vi "PicoScopeospaSetDataBuffers.vi"(5 "enabled array":i16[](array[numeric]), 7 "Buffer and Transfer Settings":T3={"startIndex"=0, "Samples"=1000, "Down Sample Ratio"=1, "Down-Sample Mode"=1} {"Down-Sample Mode" items=["RAW none"=2147483648, "None"=0, "Aggregate"=1, "Decimate"=2, "Average"=4]; "Down Sample Ratio" step=1; "Samples" format="%_6p"}, 8 "error in (no error)":errorcluster, 9 "Device Info":T1, 10 "Data Pointers In":T2={"Max Buffer Pointers"=[], "Min Buffer Pointers"=[], "StreamingDataInfo"=[[{"Channel"=0, "Down-Sample Mode"=0, "PICO_DATA_TYPE"=enum."PICO_INT16_T", "Samples"=0, "bufferIndex"=0, "startIndex"=0, "overflow"=0}]]}, 11 "handle in":i16) -> (0 "error out":errorcluster, 3 "handle out":i16)   [LabVIEW 2024]
doc: "Calls SetDataBuffers, and assigns Pico buffers"
uses:
  shared/Buffer and Transfer Settings.ctl
  shared/PicoBuffers.ctl
  psospa.dll
panel:
  out "Actionflag":bool
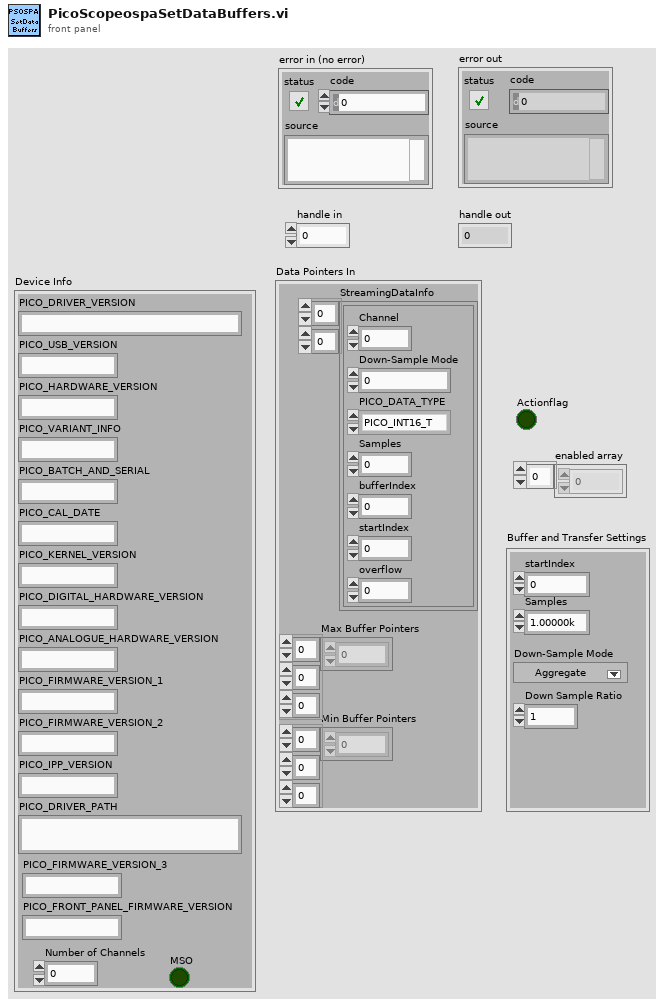
[diagram p1: front panel]
types:
  T1 = cluster{"PICO_DRIVER_VERSION":string, "PICO_USB_VERSION":string, "PICO_HARDWARE_VERSION":string, "PICO_VARIANT_INFO":string, "PICO_BATCH_AND_SERIAL":string, "PICO_CAL_DATE":string, "PICO_KERNEL_VERSION":string, "PICO_DIGITAL_HARDWARE_VERSION":string, "PICO_ANALOGUE_HARDWARE_VERSION":string, "PICO_FIRMWARE_VERSION_1":string, "PICO_FIRMWARE_VERSION_2":string, "PICO_IPP_VERSION":string, "PICO_DRIVER_PATH":string, "PICO_FIRMWARE_VERSION_3":string, "PICO_FRONT_PANEL_FIRMWARE_VERSION":string, "Number of Channels":i16, "MSO":bool}
  T2 = typedef "PicoBuffers.ctl" = cluster{"Max Buffer Pointers":u64[][][], "Min Buffer Pointers":u64[][][], "StreamingDataInfo":cluster{"Channel":u32, "Down-Sample Mode":u32, "PICO_DATA_TYPE":enum32{"PICO_INT8_T", "PICO_INT16_T", "PICO_INT32_T", "PICO_UINT32_T", "PICO_INT64_T", ""}, "Samples":i32, "bufferIndex":u64, "startIndex":i32, "overflow":i16}[][]}
  T3 = typedef "Buffer and Transfer Settings.ctl" = cluster{"startIndex":u64, "Samples":u64, "Down Sample Ratio":u64, "Down-Sample Mode":u32}
  T4 = enum32{"PICO_INT8_T", "PICO_INT16_T", "PICO_INT32_T", "PICO_UINT32_T", "PICO_INT64_T", ""}
  T5 = cluster{"status":bool, "code":u32, "source":string}
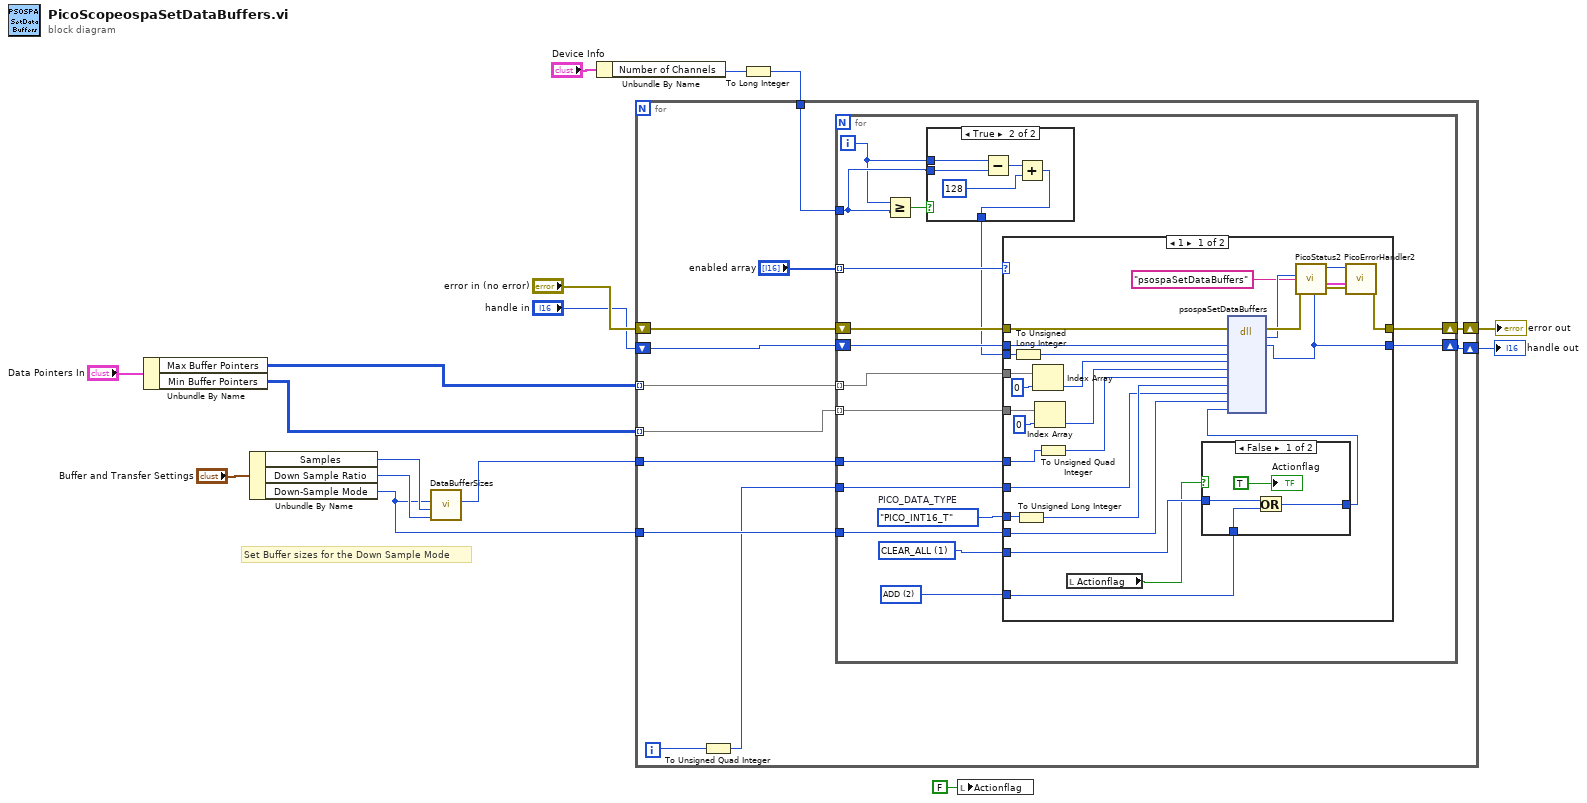
[diagram p0: block diagram]
diagram:
  # "Set Buffer sizes for the Down Sample Mode"
  n1 = Unbundle By Name("Data Pointers In") -> ("Max Buffer Pointers"=w5:u64[][][], "Min Buffer Pointers"=w4:u64[][][])
  n2 = Unbundle By Name("Buffer and Transfer Settings") -> ("Samples"=w8:u64, "Down Sample Ratio"=w9:u64, "Down-Sample Mode"=w7:u32)
  n3 = call "DataBufferSizes.vi"("Down Sample Ratio"=w9, "Number of Samples"=w8, "Down-Sample Mode"=w7) -> ("Max Buffer Size"=w10:i32)  [unwired: 7 in, 1 out]
  n4 = Unbundle By Name("Device Info") -> ("Number of Channels"=w2:i16)
  n5 = To Long Integer(number=w2) -> (32bit integer=w1:i32)
  n6 = for {
    tunnel: w10 -> [w24]
    tunnel: w7 -> [w23]
    tunnel: w5 -> [w22] mode=indexing
    tunnel: w4 -> [w21] mode=indexing
    shift-right: [w28] -> w15
    shift-left: "error in (no error)" -> [w26]
    shift-right: [w27] -> w14
    shift-left: "handle in" -> [w25]
    tunnel: w1 -> [w17]
    i -> [w18]
    n7 = To Unsigned Quad Integer(1:w18) -> (0:w19:u64)
    n8 = for {
      tunnel: w23 -> [w45]
      tunnel: w24 -> [w42]
      tunnel: "enabled array" -> [w30] mode=indexing
      tunnel: w22 -> [w41] mode=indexing
      shift-right: [w40] -> w28
      shift-left: w26 -> [w44]
      tunnel: w21 -> [w36] mode=indexing
      shift-right: [w35] -> w27
      shift-left: w25 -> [w43]
      tunnel: w19 -> [w34]
      tunnel: w17 -> [w32]
      i -> [w31]
      w37 = T4."PICO_INT16_T"  # PICO_DATA_TYPE
      w38 = u32 1 items=["NONE"=0, "CLEAR_ALL"=1, "ADD"=2, "CLEAR_THIS_DATA_BUFFER"=4096, "CLEAR_WAVEFORM_DATA_BUFFERS"=8192, "CLEAR_WAVEFORM_READ_DATA_BUFFERS"=16384] ("PicoAction 1")
      w39 = u32 2 items=["NONE"=0, "CLEAR_ALL"=1, "ADD"=2, "CLEAR_THIS_DATA_BUFFER"=4096, "CLEAR_WAVEFORM_DATA_BUFFERS"=8192, "CLEAR_WAVEFORM_READ_DATA_BUFFERS"=16384] ("PicoAction 2")
      n9 = Greater Or Equal?(x=w31, y=w32) -> (x >= y?=w33:bool)
      n10 = case shown="True" w33 {
        tunnel: [w46 w50] -> w29
        tunnel: w32 -> [_ w49]
        tunnel: w31 -> [w46 w48]
        frame False {
        }
        frame True {
          n11 = Subtract(x=w48, y=w49) -> (x-y=w47:i32)
          n12 = Add(x=w47, y=128) -> (x+y=w50:i32)
        }
      }
      n13 = case shown="1" w30 {
        tunnel: w29 -> [w67 _]
        tunnel: w44 -> [w78 w85]
        tunnel: w43 -> [w75 w84]
        tunnel: w45 -> [w72 _]
        tunnel: w37 -> [w58 _]
        tunnel: w38 -> [w62 _]
        tunnel: [w71 w85] -> w40
        tunnel: [w70 w84] -> w35
        tunnel: w42 -> [w69 _]
        tunnel: w41 -> [w63 _]
        tunnel: w39 -> [w61 _]
        tunnel: w36 -> [w55 _]
        tunnel: w34 -> [w53 _]
        frame 1 {
          n14 = To Unsigned Long Integer(number=w67) -> (unsigned 32bit integer=w66:u32)
          n15 = To Unsigned Long Integer(number=w58) -> (unsigned 32bit integer=w59:u32)
          n16 = Index Array(array=w63, index=0) -> (element=w64:u64)
          n17 = Index Array(array=w55, index=0) -> (element=w56:u64)
          n18 = To Unsigned Quad Integer(1:w69) -> (0:w68:u64)
          n19 = local read "Actionflag"() -> (w54:bool)
          n20 = case shown="False" w54 {
            tunnel: w62 -> [w82 _]
            tunnel: w61 -> [w81 w83]
            tunnel: [w80 w83] -> w60
            frame False {
              n21 = Or(x=w82, y=w81) -> (x .or. y?=w80:u32)
              "Actionflag" <- TRUE ("Actionflag")
            }
            frame True {
            }
          }
          n22 = dll-call lib="F:/Picoscope3000e/Scope_LabView/ps3000e/Treiber_und_SubVis/psospa.dll" fn="psospaSetDataBuffers" ("ps3000.dll:_ps3000_open_unit@0")(error in=w78, "handle"=w75, "channel"=w66, "bufferMax"=w64, "bufferMin"=w56, "nSamples"=w68, "dataType"=w59, "waveform"=w53, "downSampleRatioMode"=w72, "action"=w60) -> (error out=w77:errorcluster, "PICO_STATUS"=w76:u32, "handle"=w70:i16)  [unwired: 10 in, 1 out]
          n23 = call "PicoStatus2.vi"("PICO source"="psospaSetDataBuffers" ("source"), "Error in"=w77, "PICO STATUS"=w76) -> ("error out"=w73:errorcluster, "PICO_STATUS out"=w52:T5)  [unwired: 5 in]
          n24 = call "PicoErrorHandler2.vi"("error in (no error)"=w73, "PICO_STATUS in"=w52, "handle In"=w70) -> ("error out"=w71:errorcluster)  [unwired: 8 in]
        }
        frame 0, Default {
        }
      }
    }
  }
  "error out" <- w15
  "handle out" <- w14
  n25 = local write "Actionflag"(FALSE ("Actionflag")) -> ()
